vi "test_assert_same_type.vi"() -> ()   [LabVIEW 2021]
uses:
  91db3e68-2553-3fda-405c-0747459adf3f.vi
  eef6ec20-da8f-3fe8-d08c-4959302cda3f.vi
panel:
  out "output cluster":cluster{"String a":string, "String b":string}
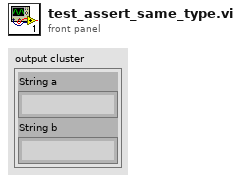
[diagram p1: front panel]
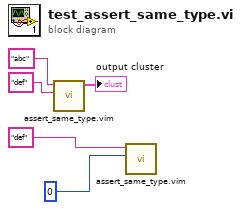
[diagram p0: block diagram]
diagram:
  n1 = call "assert_same_type.vim"("String b"="def", "String a"="abc") -> ("output cluster"=→"output cluster":cluster{"String a":string, "String b":string})  [unwired: 9 in]
  n2 = call "assert_same_type.vim"("String b"=0, "String a"="def") -> ()  [unwired: 9 in, 1 out]
